vi "Host Main.vi"() -> ()   [LabVIEW 2014]
doc: "This application launches and executes the Tag Bus Data framework configuration for the specified target alias. This is a simple example of the framework API functions, but may also be a suitable starting point for a Host UI or Thick Client that is running a local version of the framework."
uses:
  <vilib>/NI/Module Execution Interface/Engine Runtime/Execution States.ctl
  <vilib>/NI/Module Execution Interface/Engine Runtime/Fault.ctl
  <vilib>/NI/Tag Bus Module Framework/runtime/error classification.ctl
  <vilib>/NI/Current Value Table/DataTypes/I32_Read.vi
  <vilib>/NI/Current Value Table/DataTypes/I32_Write.vi
  <vilib>/NI/Current Value Table/Type to Enum.vi
  <vilib>/NI/Current Value Table/DataTypes/I32_Type To Enum.vi
  <vilib>/NI/Current Value Table/FGVs/CVT Globals.vi
  <vilib>/NI/Current Value Table/FGVs/Tag Memory.vi
  <vilib>/NI/Current Value Table/Memory Block.vi
  <vilib>/NI/Current Value Table/DataTypes/I32_Memory Block.vi
  <vilib>/userdefined/High Color/nirio_resource_hc.ctl
  <vilib>/NI/Module Execution Interface/Engine Runtime/Engine Runtime Interface.lvclass
  <vilib>/NI/DCAF/Tag Editor Core/Framework Configuration Classes/target runtime/PL_Target Runtime.lvclass
  <vilib>/NI/Tag Bus Module Framework/FPGA manager/FPGA manager.lvlib
  <vilib>/rvi/interface/nirviOpenFPGA/nirviOpenFPGA.xnode
  <vilib>/NI/Tag Bus Module Framework/FPGA manager/methods.ctl
  FPGA Module tests.lvlib
  <vilib>/NI/Current Value Table/Current Value Table.lvlib
  <vilib>/NI/Tag Bus Module Framework/runtime/TBM module execution interface.lvclass
panel:
  out "Value":i32
  in  "I32 Control":i32
  in  "configuration file path":path=path "/home/lvuser/FPGATestConfig.pcfg"
  in  "target alias":string="cRIO"
  out "engine status":T4(array[cluster])
  in  "stop":bool
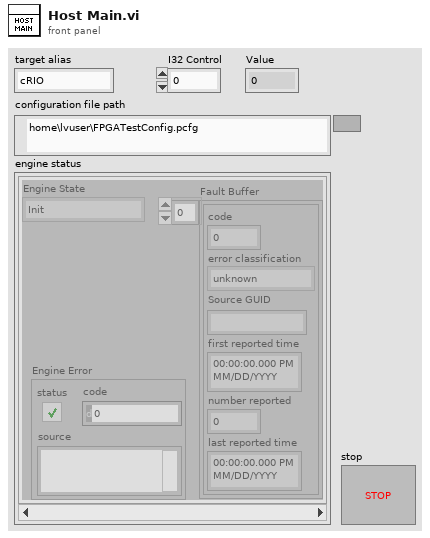
[diagram p1: front panel]
types:
  T1 = typedef "Engine Runtime Interface.lvclass/Execution States.ctl" = enum16{"Init", "Pre-Operational", "Safe-Operational", "Operational", "Stopped"}
  T2 = typedef "Engine Runtime Interface.lvclass/Fault.ctl" = cluster{"code":i32, "error classification":T3, "Source GUID":string, "first reported time":timestamp, "number reported":u32, "last reported time":timestamp}
  T3 = typedef "TBM module execution interface.lvclass/error classification.ctl" = enum16{"unknown", "none", "trivial", "recoverable", "critical"}
  T4 = cluster{"Engine State":T1, "Fault Buffer":T2[], "Engine Error":errorcluster}[]
  T5 = typedef "FPGA manager.lvlib/methods.ctl" = enum16{"initialize bitfile", "cache bitfile", "locate bitfile", "close bitfile", "clear manager"}
  T6 = typedef "nirio_resource_hc.ctl" = tag
  T7 = cluster{"Engine State":T1, "faults":T2[], "Engine Error":errorcluster}
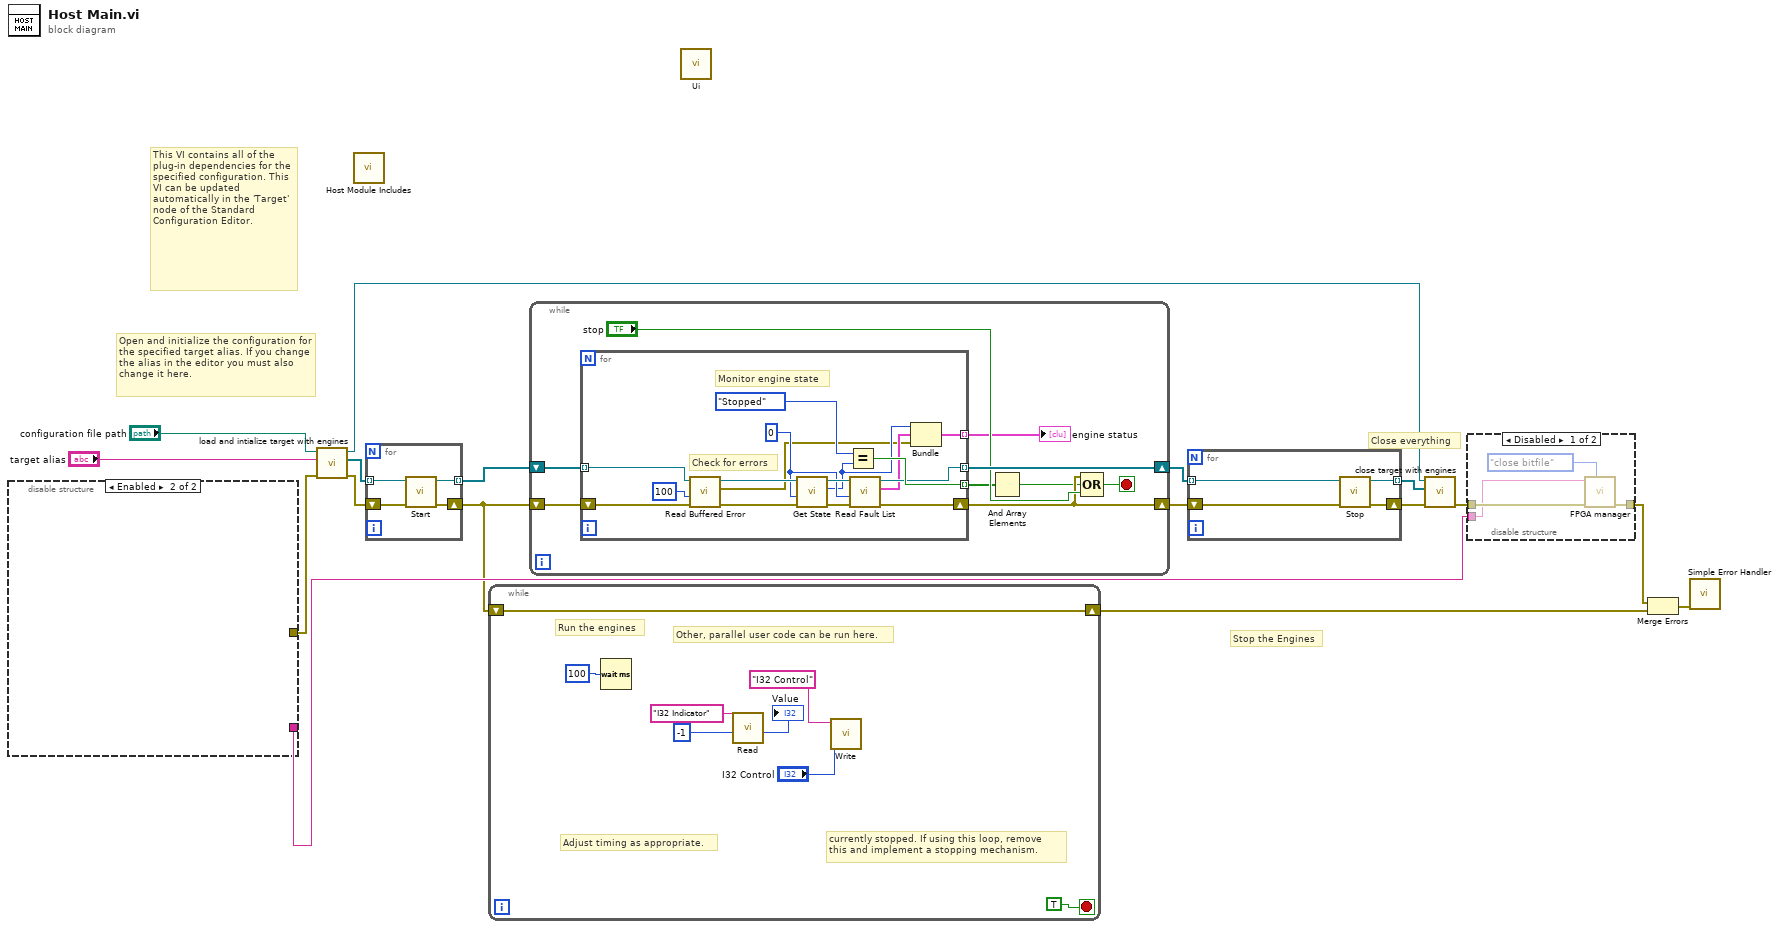
[diagram p0: block diagram]
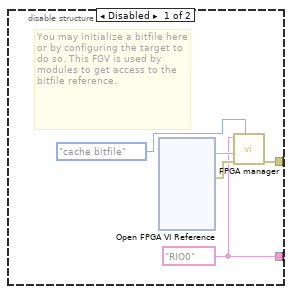
[diagram p3: hidden frame]
diagram:
  # "Open and initialize the configuration for the specified target alias. If you change the alias in the editor you must also change it here."
  # "Close everything"
  # "Stop the Engines"
  # "This VI contains all of the plug-in dependencies for the specified configuration. This VI can be updated automatically in the 'Target' node of the Standard Configuration Editor."
  # "Run the engines"
  n1 = disable-structure shown="Enabled" {
    disable-tunnel: [w22 _] -> w7
    disable-tunnel: [w18 _] -> w6
    frame Disabled {
      w18 = T6 "RIO0" ("RIO resource")
      # "You may initialize a bitfile here or by configuring the target to do so. This FGV is used by modules to get access to the bitfile reference."
      n2 = xnode "Open FPGA VI Reference"() -> ("FPGA VI Reference Out"=w20:refnum<k20>, "error out"=w21:errorcluster)  [unwired: 2 in]
      n3 = call <vilib>:"FPGA manager.vi"("action"=methods."cache bitfile", "error in"=w21, "bitfile to cache"=w20, "RIO resource"=w18) -> ("error out"=w22:errorcluster)  [unwired: 5 in, 2 out]
    }
    frame Enabled {
    }
  }
  n4 = call <vilib>:"load and intialize target with engines.vi"("error in"=w7, "target alias"="target alias", "file path"="configuration file path") -> ("error out"=w14:errorcluster, "engine runtime interfaces"=w13:refnum<class "Engine Runtime Interface.lvclass">[], "target runtime"=w10:refnum<class "PL_Target Runtime.lvclass">)  [unwired: 6 in]
  n5 = call "Host Module Includes.vi"() -> ()  [unwired: 12 in]
  n6 = for {
    tunnel: [w26] -> w17 mode=indexing
    tunnel: w13 -> [w23] mode=indexing
    shift-right: [w25] -> w5
    shift-left: w14 -> [w24]
    n7 = call-dynamic "Start.vi"("error in"=w24, "Engine Runtime Interface in"=w23) -> ("error out"=w25:errorcluster, "Engine Runtime Interface out"=w26:refnum<class "Engine Runtime Interface.lvclass">)  [unwired: 8 in]
  }
  n8 = while {
    shift-right: [w32] -> w4
    shift-left: w5 -> [w32]
    stop <- TRUE stop-if-true
    # "currently stopped. If using this loop, remove \nthis and implement a stopping mechanism."
    # "Adjust timing as appropriate."
    # "Other, parallel user code can be run here."
    n9 = Wait (ms)(milliseconds to wait=u32 100) -> ()  [unwired: 1 out]
    n10 = call-poly <vilib>:"Read.vi"("Default"=-1, "Tag Name"="I32 Indicator") -> ("Value"=→"Value":i32)  [unwired: 8 in, 1 out]
    n11 = call-poly <vilib>:"Write.vi"("Value"="I32 Control", "Tag Name"="I32 Control") -> ()  [unwired: 9 in, 1 out]
  }
  n12 = while {
    shift-right: [w41] -> w16
    shift-left: w17 -> [w43]
    shift-right: [w38] -> w15
    shift-left: w5 -> [w42]
    stop <- w39 stop-if-true
    n13 = for {
      tunnel: w43 -> [w59] mode=indexing
      tunnel: [w50] -> w41 mode=indexing
      tunnel: [w54] -> w36 mode=indexing
      shift-right: [w49] -> w38
      shift-left: w42 -> [w58]
      tunnel: [w44] -> w37 mode=indexing
      w48 = 0 ("timeout (-1)")
      # "Monitor engine state"
      # "Check for errors"
      n14 = call-dynamic "Read Buffered Error.vi"("error in"=w58, "timeout in ms (0)"=100, "Engine Runtime Interface in"=w59) -> ("error out"=w56:errorcluster, "Engine Error"=w45:errorcluster, "Engine Runtime Interface out"=w57:refnum<class "Engine Runtime Interface.lvclass">)  [unwired: 6 in]
      n15 = call-dynamic "Get State.vi"("error in"=w56, "timeout (-1)"=w48, "Engine Runtime Interface in"=w57) -> ("error out"=w52:errorcluster, "Engine State"=w47:T1, "Engine Runtime Interface out"=w51:refnum<class "Engine Runtime Interface.lvclass">)  [unwired: 6 in]
      n16 = Equal?(x=Execution_States."Stopped" ("Engine State"), y=w47) -> (x = y?=w54:bool)
      n17 = call-dynamic "Read Fault List.vi"("error in"=w52, "timeout (-1)"=w48, "Engine Runtime Interface in"=w51) -> ("error out"=w49:errorcluster, "faults"=w46:T2[], "Engine Runtime Interface out"=w50:refnum<class "Engine Runtime Interface.lvclass">)  [unwired: 6 in]
      n18 = Bundle("Engine State"=w47, "faults"=w46, "Engine Error"=w45) -> (w44:T7)  [unwired: 1 in]
    }
    "engine status" <- w37
    n19 = And Array Elements(Boolean array=w36) -> (logical AND=w35:bool)
    n20 = Compound Arithmetic op=OR(w38, w35, "stop") -> (w39:bool)
  }
  n21 = call "Ui.vi"() -> ()  [unwired: 12 in]
  n22 = for {
    tunnel: w16 -> [w63] mode=indexing
    shift-right: [w60] -> w9
    shift-left: w15 -> [w62]
    tunnel: [w61] -> w11 mode=indexing
    n23 = call-dynamic "Stop.vi"("error in"=w62, "Engine Runtime Interface in"=w63) -> ("error out"=w60:errorcluster, "Engine Runtime Interface out"=w61:refnum<class "Engine Runtime Interface.lvclass">)  [unwired: 8 in]
  }
  n24 = call <vilib>:"close target with engines.vi"("error in"=w9, "Engine Runtime Interfaces"=w11, "Target Runtime"=w10) -> ("error out"=w3:errorcluster)  [unwired: 8 in]
  n25 = disable-structure shown="Disabled" {
    disable-tunnel: [w66 w68] -> w2
    disable-tunnel: w3 -> [w67 w68]
    disable-tunnel: w6 -> [w64 _]
    frame Disabled {
      n26 = call <vilib>:"FPGA manager.vi"("action"=methods."close bitfile", "error in"=w67, "RIO resource"=w64) -> ("error out"=w66:errorcluster)  [unwired: 6 in, 2 out]
    }
    frame Enabled {
    }
  }
  n27 = Merge Errors(w2, w4) -> (w1:errorcluster)
  n28 = call <vilib>:"Simple Error Handler.vi"("error in (no error)"=w1) -> ()  [unwired: 4 in, 5 out]
